vi "NISE.Get Chassis List.vi"(0 "SLSC Interface in":refnum<class "SLSC Interface.lvclass">, 11 "error in (no error)":errorcluster) -> (4 "SLSC Interface out":refnum<class "SLSC Interface.lvclass">, 8 "Sys.Chassis":refnum<k21>[](array[refnum]), 15 "error out":errorcluster)   [LabVIEW 2016, in "SLSC Interface.lvclass"]
uses:
  SLSC Interface.lvclass
  SLSC Interface.lvclass/SLSC Interface.ctl
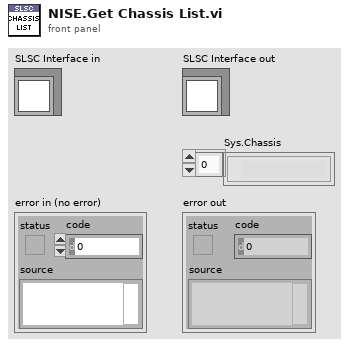
[diagram p1: front panel]
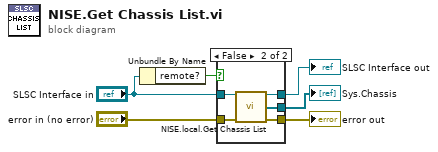
[diagram p0: block diagram]
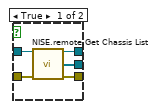
[diagram p2: hidden frame]
diagram:
  n1 = Unbundle By Name("SLSC Interface in") -> ("remote?"=w6:bool)
  n2 = case shown="False" w6 {
    tunnel: "SLSC Interface in" -> [w11 w16]
    tunnel: [w10 w15] -> w5
    tunnel: [w9 w14] -> w4
    tunnel: "error in (no error)" -> [w8 w13]
    tunnel: [w7 w12] -> w2
    frame True {
      n3 = call "NISE.remote.Get Chassis List.vi"("SLSC Remote in"=w11, "error in (no error)"=w8) -> ("SLSC Remote out"=w10:refnum<class "SLSC Interface.lvclass">, "Sys.Chassis"=w9:refnum<k21>[], "error out"=w7:errorcluster)  [unwired: 11 in]
    }
    frame False {
      n4 = call "NISE.local.Get Chassis List.vi"("SLSC Local in"=w16, "error in (no error)"=w13) -> ("SLSC Local out"=w15:refnum<class "SLSC Interface.lvclass">, "Sys.Chassis"=w14:refnum<k21>[], "error out"=w12:errorcluster)  [unwired: 11 in]
    }
  }
  "error out" <- w2
  "SLSC Interface out" <- w5
  "Sys.Chassis" <- w4
